vi "CommInitialize.vi"(8 "error in (no error)":errorcluster, 11 "Categories in":refnum<class "Categories.lvclass">) -> (0 "error out":errorcluster, 3 "Node*":refnum<data-value>)   [LabVIEW 2013, in "Categories.lvclass"]
uses:
  Categories.lvclass
  xCE/xceNode/xceNode.lvclass
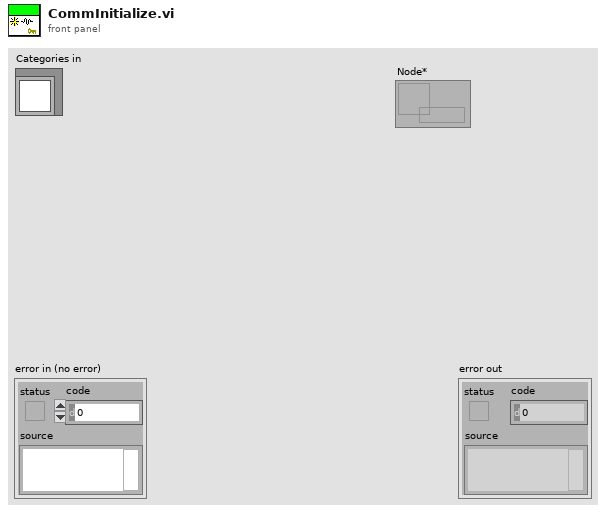
[diagram p1: front panel]
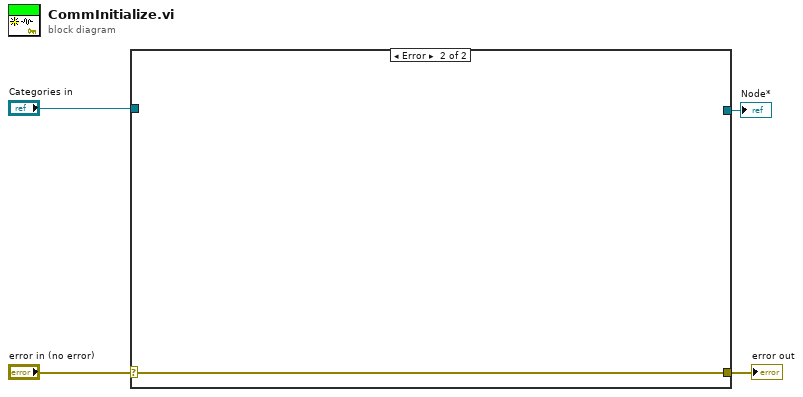
[diagram p0: block diagram]
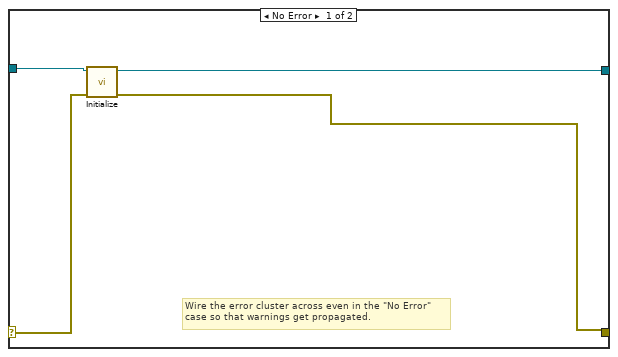
[diagram p2: hidden frame]
diagram:
  n1 = case shown="Error" "error in (no error)" {
    selector: "error in (no error)" -> [w7 w9]
    tunnel: [w5 w9] -> w4
    tunnel: "Categories in" -> [w8 _]
    tunnel: [w6 _] -> w1
    frame No Error {
      # "Wire the error cluster across even in the \"No Error\"\ncase so that warnings get propagated."
      n2 = call-dynamic "Initialize.vi"("error in"=w7, "Categories in"=w8) -> ("error out"=w5:errorcluster, "Node*"=w6:refnum<data-value>)  [unwired: 8 in]
    }
    frame Error {
    }
  }
  "error out" <- w4
  "Node*" <- w1
